vi "DAC Run.vi"(8 "error in":errorcluster, 11 "DAC DC Supply in":refnum<class "DAC DC Supply.lvclass">) -> (0 "error out":errorcluster, 3 "DAC DC Supply out":refnum<class "DAC DC Supply.lvclass">)   [LabVIEW 2019, in "DAC.lvlib" / "DAC DC Supply.lvclass"]
uses:
  DAC DC Supply.lvclass
  DAC.lvclass
  Results/Results Method.ctl
  Results/Results.lvlib
  Results/HTS Results/HTS Results.lvclass
  C:/Users/krio/Documents/LV_Projects/test-stand/App/DAC/DAC.lvclass
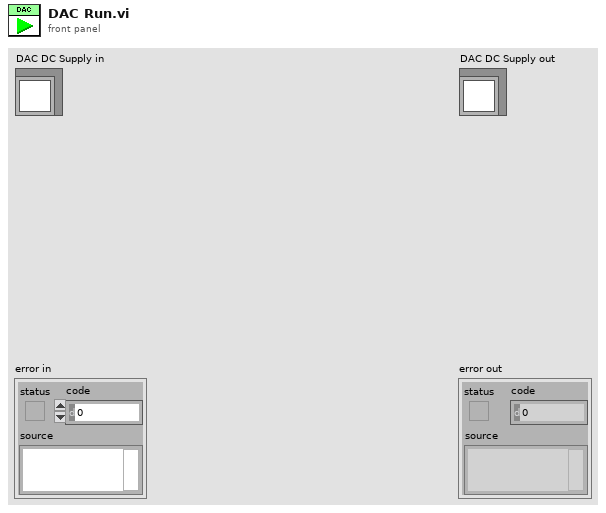
[diagram p1: front panel]
types:
  T1 = typedef "Results.lvlib/Results Method.ctl" = enum16{"Get", "Set"}
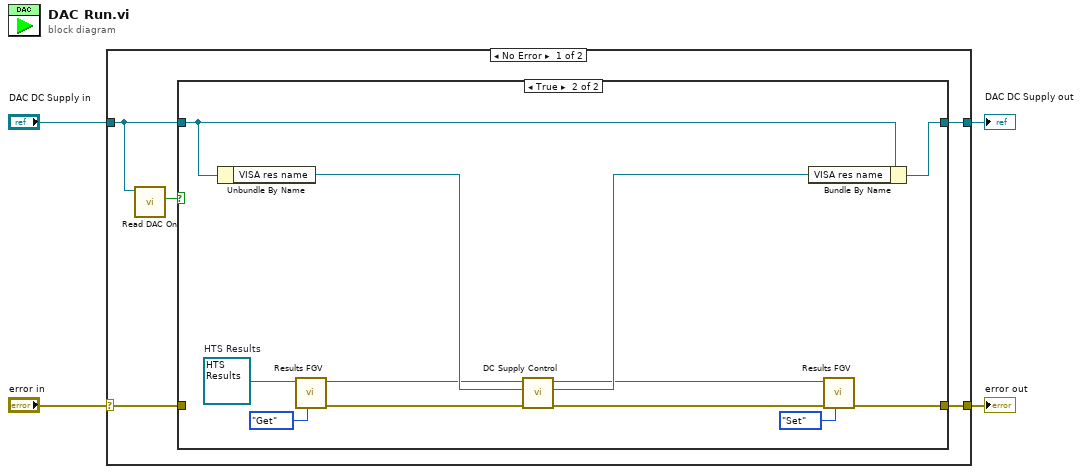
[diagram p0: block diagram]
diagram:
  n1 = case shown="No Error" "error in" {
    selector: "error in" -> [w7 w25]
    tunnel: [w6 w25] -> w2
    tunnel: [w8 w24] -> w1
    tunnel: "DAC DC Supply in" -> [w5 w24]
    frame No Error {
      n2 = call "Read DAC On.vi"("DAC in"=w5) -> ("DAC On"=w9:bool)  [unwired: 8 in, 2 out]
      n3 = case shown="True" w9 {
        tunnel: w5 -> [w11 w23]
        tunnel: [w11 w21] -> w8
        tunnel: w7 -> [w10 _]
        tunnel: [w10 w18] -> w6
        frame False {
        }
        frame True {
          w20 = refnum<class "HTS Results.lvclass"> refnum  # HTS Results
          n4 = Unbundle By Name(w23) -> ("VISA res name"=w17:refnum<visa-resource-name>)
          n5 = call-dynamic "Results FGV.vi"("Method"=Results_Method."Get", "HTS Results in"=w20) -> ("error out"=w13:errorcluster, "HTS Results out"=w15:refnum<class "HTS Results.lvclass">)  [unwired: 8 in]
          n6 = call "DC Supply Control.vi"("error in"=w13, "VISA res in"=w17, "HTS Results in"=w15) -> ("error out"=w12:errorcluster, "VISA res out"=w16:refnum<visa-resource-name>, "HTS Results out"=w14:refnum<class "HTS Results.lvclass">)  [unwired: 6 in]
          n7 = Bundle By Name(cluster=w23, "VISA res name"=w16) -> (w21:refnum<class "DAC DC Supply.lvclass">)
          n8 = call-dynamic "Results FGV.vi"("Method"=Results_Method."Set", "error in"=w12, "HTS Results in"=w14) -> ("error out"=w18:errorcluster)  [unwired: 7 in, 1 out]
        }
      }
    }
    frame Error {
    }
  }
  "error out" <- w2
  "DAC DC Supply out" <- w1
